vi "vicrypt_receiver.vi"() -> ()   [LabVIEW 2017]
panel:
  in  "JSON DATA":string
  in  "Encrypted key":string
  in  "Own modulo":string
  in  "Own private key":string
  in  "Encrypted text":string
  out "Plaintext":string
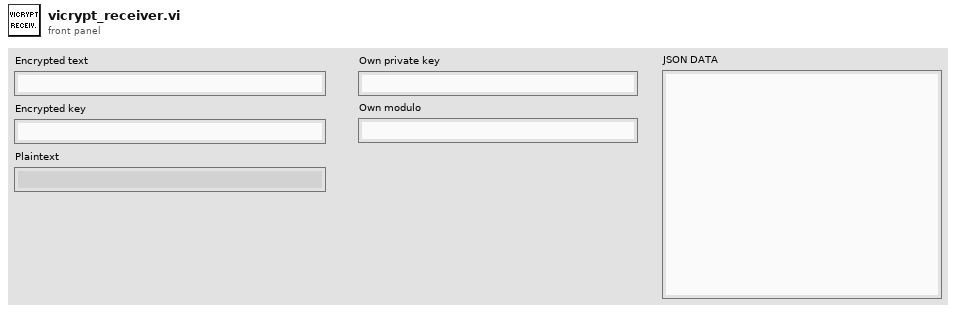
[diagram p1: front panel]
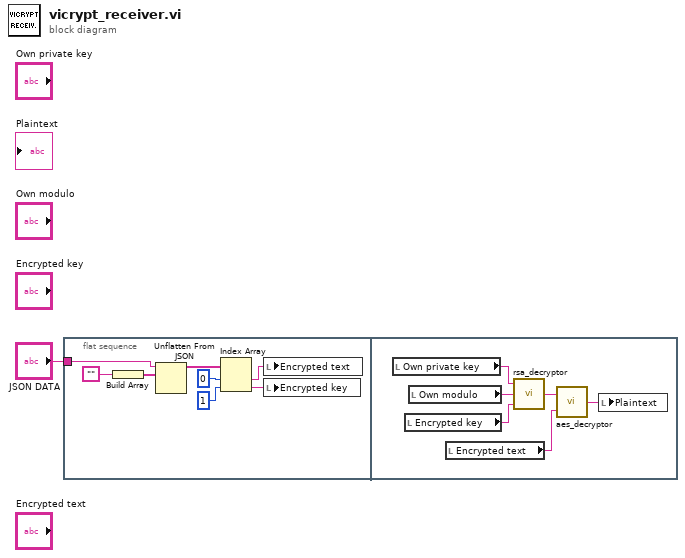
[diagram p0: block diagram]
diagram:
  n1 = flat-sequence {
    tunnel: "JSON DATA" -> [w7]
    frame #0 {
      n2 = Build Array("") -> (w9:string[])
      n3 = Unflatten From JSON(JSON string=w7, type and defaults=w9) -> (value=w4:string[])  [unwired: 5 in, 1 out]
      n4 = Index Array(array=w4, index #1=0 ("index"), index #2=1 ("index")) -> (element #1=w5:string, element #2=w2:string)
      n5 = local write "Encrypted text"(w5) -> ()
      n6 = local write "Encrypted key"(w2) -> ()
    }
    frame #1 {
      n7 = local read "Own private key"() -> (w14:string)
      n8 = local read "Encrypted key"() -> (w13:string)
      n9 = local read "Own modulo"() -> (w15:string)
      n10 = local read "Encrypted text"() -> (w10:string)
      n11 = call "rsa_decryptor.vi"("Encrypted text"=w13, "Own module"=w15, "Own private key"=w14) -> ("Decrypted text"=w12:string)
      n12 = call "aes_decryptor.vi"("Encrypted"=w10, "Key"=w12) -> ("Decrypted"=w11:string)
      n13 = local write "Plaintext"(w11) -> ()
    }
  }
